vi "Pre_Configuration_Tomography_v1.vi"(8 "error in":errorcluster, 10 "Config files paths":T4={"ZI config file (.ini)"="Tomography_v1_config_dir\\Zurich_params.ini", "Keithley config file (.ini)"="Tomography_v1_config_dir\\Keithley_params.ini", "Arduino config file (.ini)"="Tomography_v1_config_dir\\pulses_sequence_dir"}, 11 "Resources in":T1 {"ZI ModHandle"."ModHandle" format="0x%08x"; "ZI ModHandle"."Conn" format="0x%08x"; "ZI Handle"."Handle" format="0x%08x"; "ZI Handle"."Conn" format="0x%08x"}) -> (0 "error out":errorcluster, 3 "Resources out":T1 {"ZI ModHandle"."ModHandle" format="0x%08x"; "ZI ModHandle"."Conn" format="0x%08x"; "ZI Handle"."Handle" format="0x%08x"; "ZI Handle"."Conn" format="0x%08x"})   [LabVIEW 2021]
uses:
  Ver_1/Resources.ctl
  <instrlib>/Zurich Instruments LabOne/Public/ziTypeHandle.ctl
  <instrlib>/Zurich Instruments LabOne/Public/Modules/ziTypeModHandle.ctl
  Ver_1/Config_File_Paths.ctl
  <instrlib>/Zurich Instruments LabOne/Zurich Instruments LabOne.lvlib
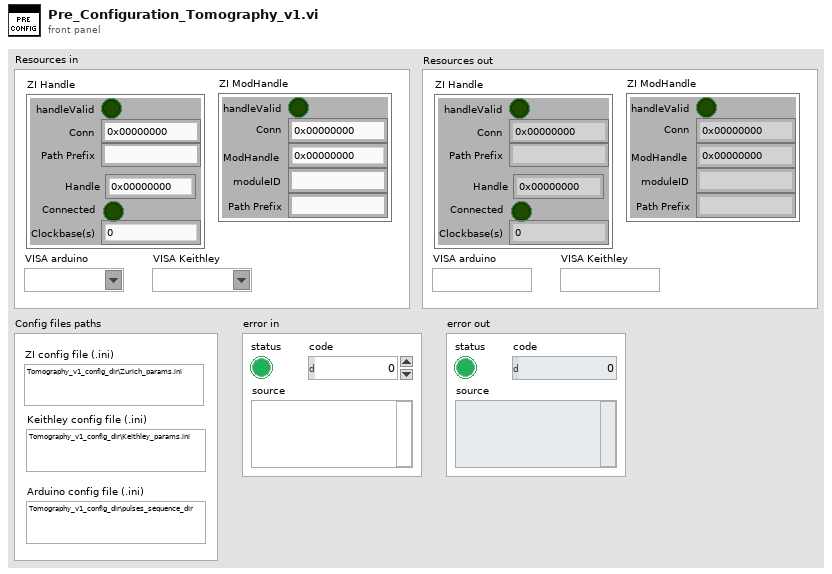
[diagram p1: front panel]
types:
  T1 = typedef "Resources.ctl" = cluster{"ZI Handle":T2, "ZI ModHandle":T3, "VISA arduino":refnum<visa-resource-name>, "VISA Keithley":refnum<visa-resource-name>}
  T2 = typedef "Zurich Instruments LabOne.lvlib/ziTypeHandle.ctl" = cluster{"handleValid":bool, "Conn":u64, "Path Prefix":string, "Handle":u64, "Connected":bool, "Clockbase(s)":dbl}
  T3 = typedef "Zurich Instruments LabOne.lvlib/ziTypeModHandle.ctl" = cluster{"handleValid":bool, "Conn":u64, "ModHandle":u64, "moduleID":string, "Path Prefix":string}
  T4 = typedef "Config_File_Paths.ctl" = cluster{"ZI config file (.ini)":string, "Keithley config file (.ini)":string, "Arduino config file (.ini)":string}
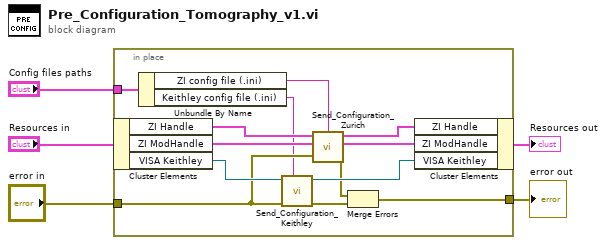
[diagram p0: block diagram]
diagram:
  n1 = in-place {
    in-place-border: "error in" -> [w12]
    in-place-border: [w9] -> w3
    in-place-border: "Config files paths" -> [w8]
    n2 = in-place-cluster #1("Resources in") -> ("ZI Handle"=w18:T2, "ZI ModHandle"=w16:T3, "VISA Keithley"=w14:refnum<visa-resource-name>)
    n3 = Unbundle By Name(w8) -> ("ZI config file (.ini)"=w7:string, "Keithley config file (.ini)"=w6:string)
    n4 = call "Send_Configuration_Keithley.vi"("Filename (.ini)"=w6, "error in"=w12, "Keithley VISA in"=w14) -> ("error out"=w10:errorcluster, "Keithley VISA out"=w13:refnum<visa-resource-name>)  [unwired: 4 in, 3 out]
    n5 = call "Send_Configuration_Zurich.vi"("Filename (.ini)"=w7, "Handle In"=w18, "ModHandle In"=w16, "error in"=w12) -> ("Handle Out"=w17:T2, "ModHandle Out"=w15:T3, "error out"=w11:errorcluster)  [unwired: 1 in]
    n6 = Merge Errors(w11, w10) -> (w9:errorcluster)
    n7 = in-place-cluster #1("ZI Handle"=w17, "ZI ModHandle"=w15, "VISA Keithley"=w13) -> (→"Resources out":T1)
  }
  "error out" <- w3
